vi "Get Queue Status.vi"(8 "error in (no error)":errorcluster, 11 "Priority Queue In":T1) -> (0 "error out":errorcluster, 1 "# Pending Insert":i32, 2 "# Pending Remove":i32, 3 "Priority Queue Out":T1, 4 "# Elements In Queue":i32)   [LabVIEW 2017, in "Communicable State Machine.lvlib"]
doc: "### Get Queue Status.vi\n\n-- <b>Controls</b> --\n- <b>Priority Queue in</b>:\n\n-- <b>Indicators</b> --\n- <b># pending insert</b>:\n- <b># pending remove</b>:\n- <b>Priority Queue out</b>:\n- <b># elements in queue</b>:"
uses:
  Communicable State Machine.lvlib
  Priority Queue.ctl
  Typedef/_Cross CSM State Data.ctl
  Typedef/_CSM_MSG_TYPE.ctl
  Typedef/_Cross CSM State Response.ctl
  Typedef/_CSM_Response Source Message.ctl
  def-Data(LowPRI-Q).ctl
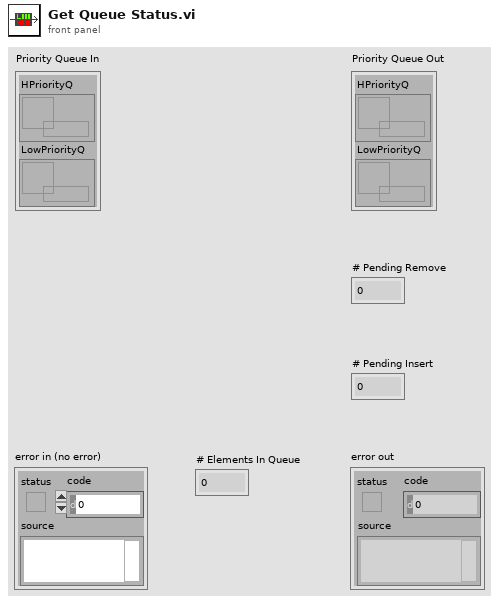
[diagram p1: front panel]
types:
  T1 = typedef "Communicable State Machine.lvlib/Priority Queue.ctl" = cluster{"HPriorityQ":refnum<queue>, "LowPriorityQ":refnum<queue>}
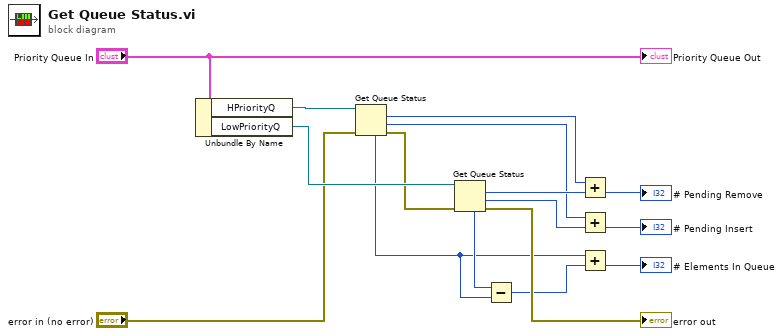
[diagram p0: block diagram]
diagram:
  n1 = Unbundle By Name("Priority Queue In") -> ("HPriorityQ"=w15:refnum<queue>, "LowPriorityQ"=w14:refnum<queue>)
  n2 = Get Queue Status(queue=w15, error in (no error)="error in (no error)") -> (# pending remove=w5:i32, # pending insert=w4:i32, error out=w11:errorcluster, # elements in queue=w2:i32)  [unwired: 1 in, 4 out]
  n3 = Get Queue Status(queue=w14, error in (no error)=w11) -> (# pending remove=w13:i32, # pending insert=w12:i32, error out=→"error out":errorcluster, # elements in queue=w3:i32)  [unwired: 1 in, 4 out]
  n4 = Subtract(x=w3, y=w2) -> (x-y=w1:i32)
  n5 = Add(x=w5, y=w13) -> (x+y=→"# Pending Remove":i32)
  n6 = Add(x=w4, y=w12) -> (x+y=→"# Pending Insert":i32)
  n7 = Add(x=w2, y=w1) -> (x+y=→"# Elements In Queue":i32)
  "Priority Queue Out" <- "Priority Queue In"
